vi "Create Sessions.vi"(7 "require single session":bool, 8 "error in":errorcluster, 9 "instrument":refnum<class "IInstrument.lvclass">, 10 "data in":T1, 11 "state in":refnum<class "Reserved State.lvclass">) -> (0 "error out":errorcluster, 1 "sessions":variant[](array[variant]), 2 "data out":T1, 4 "channel lists":string[](array[string]))   [LabVIEW 2020, in "MeasurementLink Session Management.lvlib" / "Reserved State.lvclass"]
uses:
  Reserved State.lvclass
  Reserved State.lvclass/Reserved State.ctl
  Session Reservation/Session Reservation.lvclass
  IState/IState.lvclass
  MeasurementLink Session Management Client/RPC Messages/ni_measurementlink_sessionmanagement_v1_ChannelMapping.ctl
  MeasurementLink Session Management Client/MeasurementLink Session Management Client.lvlib
  MeasurementLink Session Management Client/RPC Messages/nidevice_grpc_Session.ctl
  MeasurementLink Session Management Client/RPC Messages/ni_measurementlink_sessionmanagement_v1_SessionInformation.ctl
  MeasurementLink Instrument/IInstrument/IInstrument.lvclass
  Session Reservation/Session and Driver Info.ctl
  MeasurementLink Session Management Client/RPC Messages/ni_measurementlink_PinMapContext.ctl
  Connection Map/Connection Map.lvclass
  Session Reservation/Data.ctl
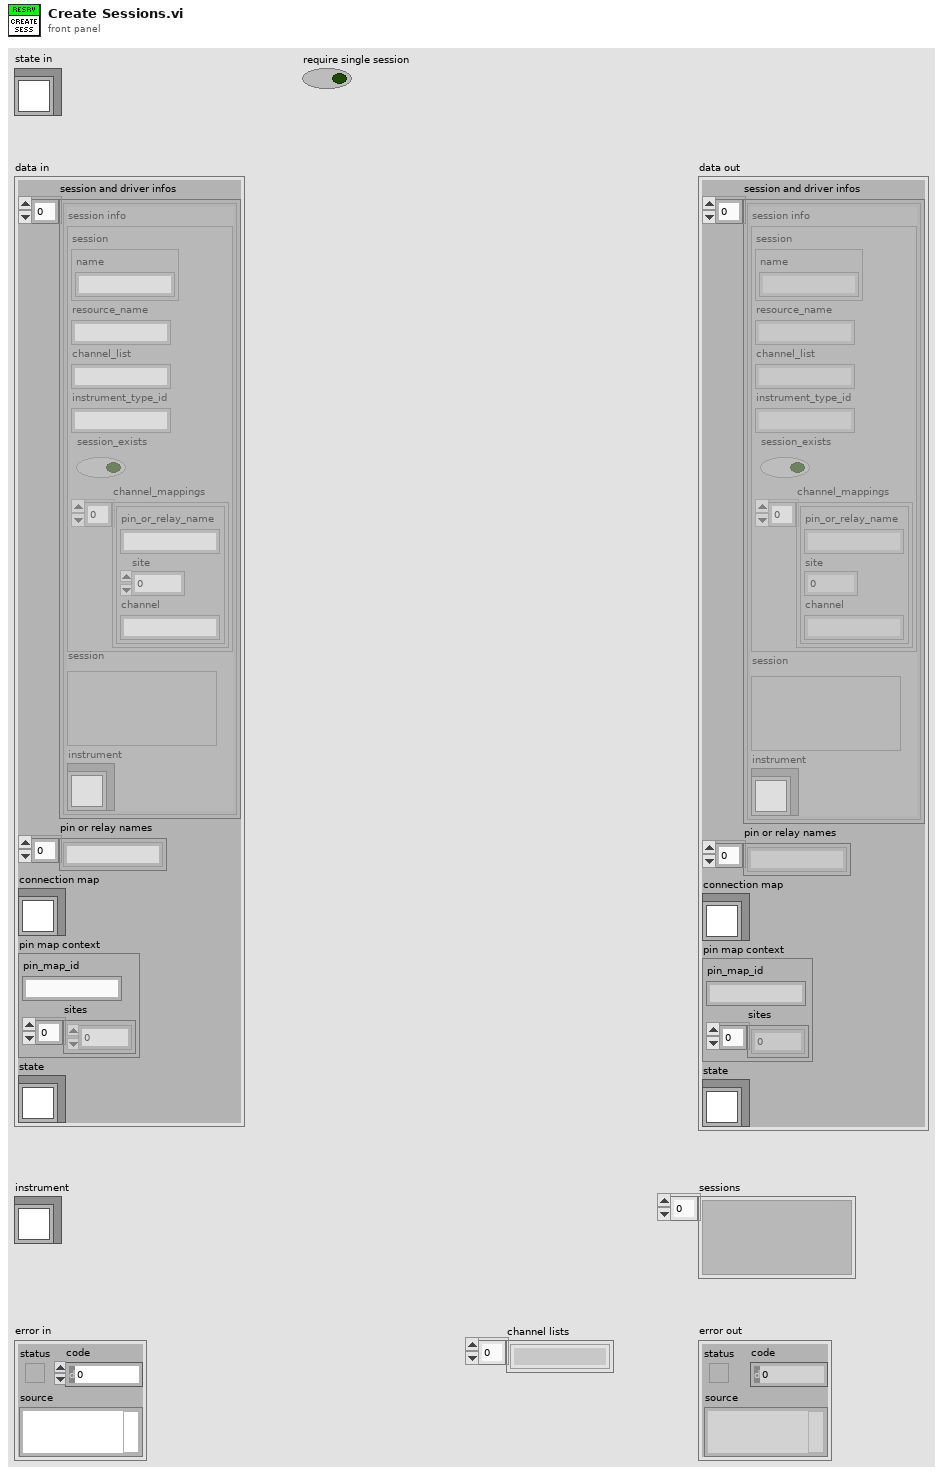
[diagram p1: front panel]
types:
  T1 = typedef "MeasurementLink Session Management.lvlib/Session Reservation.lvclass/Data.ctl" = cluster{"session and driver infos":T2[], "pin or relay names":string[], "connection map":refnum<class "Connection Map.lvclass">, "pin map context":T6, "state":refnum<class "IState.lvclass">}
  T2 = typedef "MeasurementLink Session Management.lvlib/Session Reservation.lvclass/Session and Driver Info.ctl" = cluster{"session info":T3, "session":variant, "instrument":refnum<class "IInstrument.lvclass">}
  T3 = typedef "MeasurementLink Session Management Client.lvlib/ni_measurementlink_sessionmanagement_v1_SessionInformation.ctl" = cluster{"session":T4, "resource_name":string, "channel_list":string, "instrument_type_id":string, "session_exists":bool, "channel_mappings":T5[]}
  T4 = typedef "MeasurementLink Session Management Client.lvlib/nidevice_grpc_Session.ctl" = cluster{"name":string}
  T5 = typedef "MeasurementLink Session Management Client.lvlib/ni_measurementlink_sessionmanagement_v1_ChannelMapping.ctl" = cluster{"pin_or_relay_name":string, "site":i32, "channel":string}
  T6 = typedef "MeasurementLink Session Management Client.lvlib/ni_measurementlink_PinMapContext.ctl" = cluster{"pin_map_id":string, "sites":i32[]}
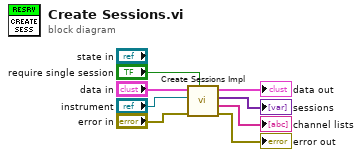
[diagram p0: block diagram]
diagram:
  n1 = call "Create Sessions Impl.vi"("require single session"="require single session", "error in"="error in", "instrument"="instrument", "data in"="data in") -> ("error out"=→"error out":errorcluster, "channel lists"=→"channel lists":string[], "sessions"=→"sessions":variant[], "data out"=→"data out":T1)  [unwired: 4 in]
